vi "ParseCurrentPVResponce.vi"() -> ()   [LabVIEW 2017]
panel:
  in  "Responce":u8[](array[numeric])=[2, 48, 49, 65, 77, 73, 44, 79, 75, 44, 84, 69, 77, 80, 45, 50, 48, 48, 48, 32, 32, 86, 48, 48, 45, 82, 48, 48, 50, 52, 13, 10] format="%x"
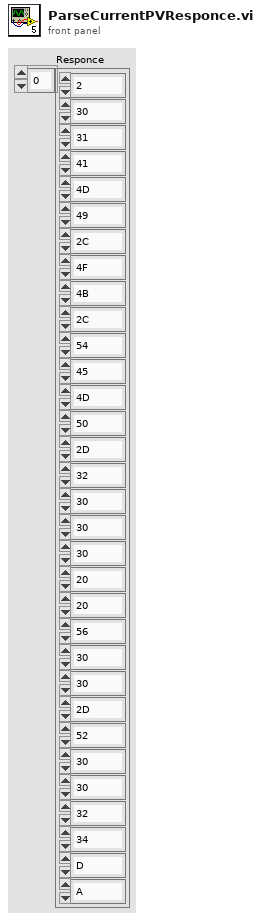
[diagram p1: front panel]
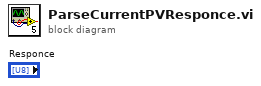
[diagram p0: block diagram]
diagram:
